vi "DIO_I2C.vi"(0 "DIO.1:0.OUT":fxp<+,2,2> format="%02b", 1 "DIO.1:0.DIR":fxp<+,2,2> format="%02b", 2 "I2C.CNFG":u8, 3 "I2C.CNTL":u8, 4 "I2C.ADDR":u8, 5 "I2C.DATO":u8, 6 "DIO.1/I2C.SDA":refnum<k21>, 7 "I2C.CNTR":u8=187, 8 "DIO.0/I2C.SCL":refnum<k21>, 9 "Execute?":T1, 11 "SELECT":bool) -> (14 "DIO.1:0.IN":fxp<+,2,2> format="%02b", 18 "I2C.DATI":u8, 19 "I2C.STAT":u8)   [LabVIEW 2013]
uses:
  Utilities/Start Boolean.ctl
  <vilib>/rvi/eio/common/nirviEmuTemplateMethod_errors.vi
  <vilib>/eio/EIONode/EIONode.xnode
panel:
  # "SELECT | Functionality \n --------|-------------\n     0   | DIO0, DIO1\n     1   | I2C: SDA, SCL"
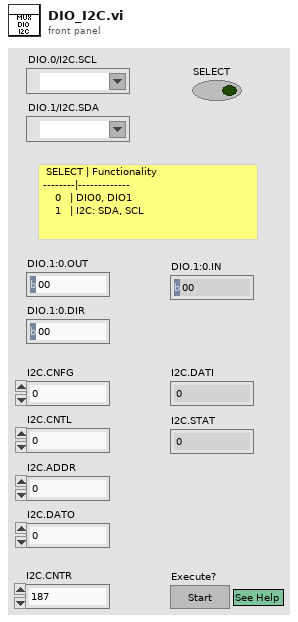
[diagram p1: front panel]
types:
  T1 = typedef "Start Boolean.ctl" = bool
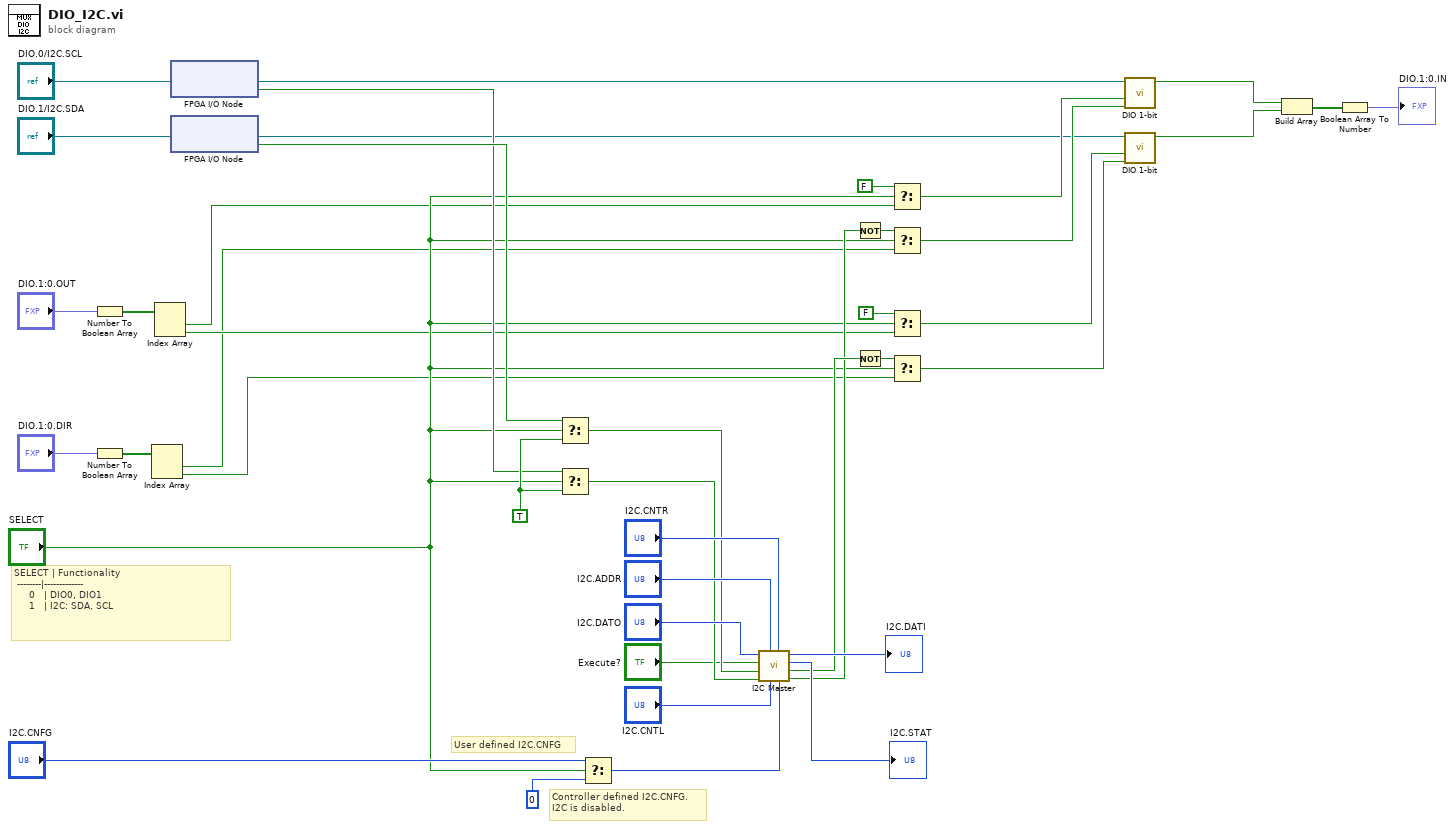
[diagram p0: block diagram]
diagram:
  w30 = TRUE ("f")
  # "Controller defined I2C.CNFG.\nI2C is disabled."
  # "User defined I2C.CNFG"
  # "SELECT | Functionality \n --------|-------------\n     0   | DIO0, DIO1\n     1   | I2C: SDA, SCL"
  n1 = Number To Boolean Array(number="DIO.1:0.OUT") -> (Boolean array=w20:bool[])
  n2 = Number To Boolean Array(number="DIO.1:0.DIR") -> (Boolean array=w19:bool[])
  n3 = Index Array(array=w19) -> (element #1=w1:bool, element #2=w2:bool)  [unwired: 2 in]
  n4 = Index Array(array=w20) -> (element #1=w4:bool, element #2=w3:bool)  [unwired: 2 in]
  n5 = xnode "FPGA I/O Node"("FPGA I/O In"="DIO.0/I2C.SCL") -> ("I/O Item"=w13:bool, "FPGA I/O Out"=w11:refnum<k21>)
  n6 = xnode "FPGA I/O Node"("FPGA I/O In"="DIO.1/I2C.SDA") -> ("I/O Item"=w15:bool, "FPGA I/O Out"=w12:refnum<k21>)
  n7 = Select(t=w15, s="SELECT", f=w30) -> (s? t:f=w32:bool)
  n8 = Select(t=w13, s="SELECT", f=w30) -> (s? t:f=w33:bool)
  n9 = Select(t="I2C.CNFG", s="SELECT", f=u8 0) -> (s? t:f=w34:u8)
  n10 = call "I2C Master.vi"("Configuration"=w34, "Counter"="I2C.CNTR", "Control"="I2C.CNTL", "Address In"="I2C.ADDR", "SCL_IN"=w33, "SDA_IN"=w32, "Execute?"="Execute?", "Data Out"="I2C.DATO") -> ("SCL_OUT"=w29:bool, "SDA_OUT"=w31:bool, "Status"=→"I2C.STAT":u8, "Data In"=→"I2C.DATI":u8)
  n11 = Not(x=w29) -> (.not. x?=w7:bool)
  n12 = Not(x=w31) -> (.not. x?=w8:bool)
  n13 = Select(t=FALSE, s="SELECT", f=w4) -> (s? t:f=w24:bool)
  n14 = Select(t=w7, s="SELECT", f=w1) -> (s? t:f=w23:bool)
  n15 = Select(t=FALSE ("PORTx"), s="SELECT", f=w3) -> (s? t:f=w26:bool)
  n16 = Select(t=w8, s="SELECT", f=w2) -> (s? t:f=w25:bool)
  n17 = call "DIO 1-bit.vi"("DIR"=w23, "OUT"=w24, "DIO Refnum"=w11) -> ("IN"=w6:bool)  [unwired: 8 in]
  n18 = call "DIO 1-bit.vi"("DIR"=w25, "OUT"=w26, "DIO Refnum"=w12) -> ("IN"=w5:bool)  [unwired: 8 in]
  n19 = Build Array(w6, w5) -> (w18:bool[])
  n20 = Boolean Array To Number(Boolean array=w18) -> (number=→"DIO.1:0.IN":fxp<+,2,2>)
